vi "Trim Unnecessary Zeros of Numeric String.vi"(11 "float String":string) -> (3 "float String without unnccessary zeros":string)   [LabVIEW 2017]
doc: "Removes trailing zeros, and a trailing decimal point, from a floating-point number formatted as a string."
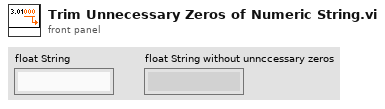
[diagram p1: front panel]
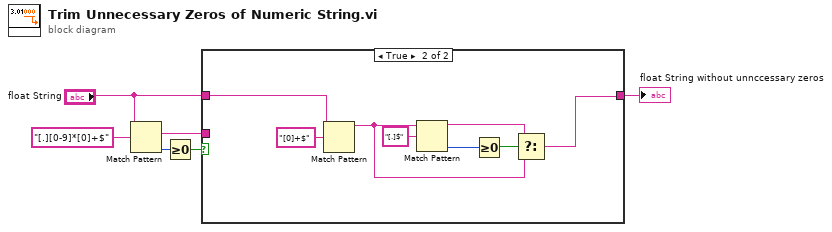
[diagram p0: block diagram]
diagram:
  n1 = Match Pattern(string="float String", regular expression="[.][0-9]*[0]+$") -> (match substring=w5:string, offset past match=w2:i32)  [unwired: 1 in, 2 out]
  n2 = Greater Or Equal To 0?(x=w2) -> (x >= 0?=w3:bool)
  n3 = case shown="True" w3 {
    tunnel: [w7 w15] -> w6
    tunnel: "float String" -> [w7 w13]
    tunnel: w5 -> [_ _]
    frame False {
    }
    frame True {
      n4 = Match Pattern(string=w13, regular expression="[0]+$") -> (before substring=w12:string)  [unwired: 1 in, 3 out]
      n5 = Match Pattern(string=w12, regular expression="[.]$") -> (before substring=w8:string, offset past match=w10:i32)  [unwired: 1 in, 2 out]
      n6 = Greater Or Equal To 0?(x=w10) -> (x >= 0?=w9:bool)
      n7 = Select(t=w8, s=w9, f=w12) -> (s? t:f=w15:string)
    }
  }
  "float String without unnccessary zeros" <- w6
